vi "LHF.DB.Mongo.Collection.Update.vi"(6 "Query":variant, 8 "error in (no error)":errorcluster, 9 "Update":variant, 10 "Collection":string, 11 "LHF.DB.Mongo in":refnum<class "LHF.DB.Mongo.lvclass">) -> (0 "error out":errorcluster, 1 "DocumentsAffected":i64, 2 "Ok":bool, 3 "LHF.DB.Mongo out":refnum<class "LHF.DB.Mongo.lvclass">)   [LabVIEW 2013, in "LHF.DB.Mongo.lvclass"]
doc: "Update: wire cluster of elements to be updated, use element name to choose database field to update. If a single field being updated you may name the variable name as the desired field to be updated.\nQuery: use clusters named with query operation (if none, equal is used) or a Query.NET object. If a single field is being queried, you may it by setting the variable name as the field name in database. \nYou may use <, <=, >, >=, ==, !=, and others in variables name to choose operation, and you may aggregate them by putting in a cluster with $and or $or."
uses:
  LHF.DB.Mongo.lvclass
  C:/Users/Ricardo/Desktop/Projetos/LabVIEW-MongoDB/src/Driver/MongoDB.Driver.dll
  LabVIEW-MongoDB/src/Driver/MongoDB.Driver.dll
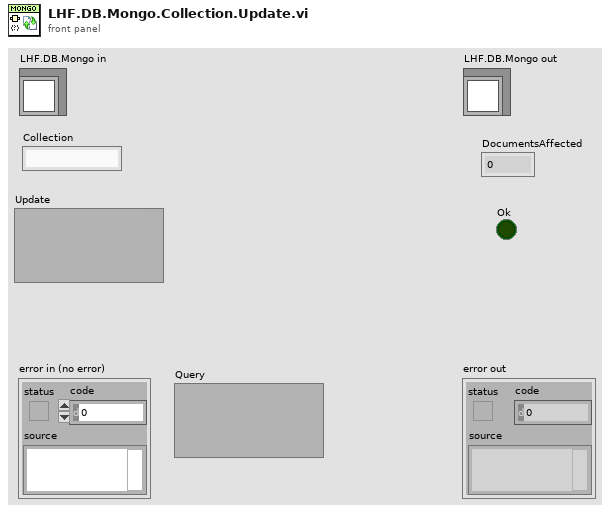
[diagram p1: front panel]
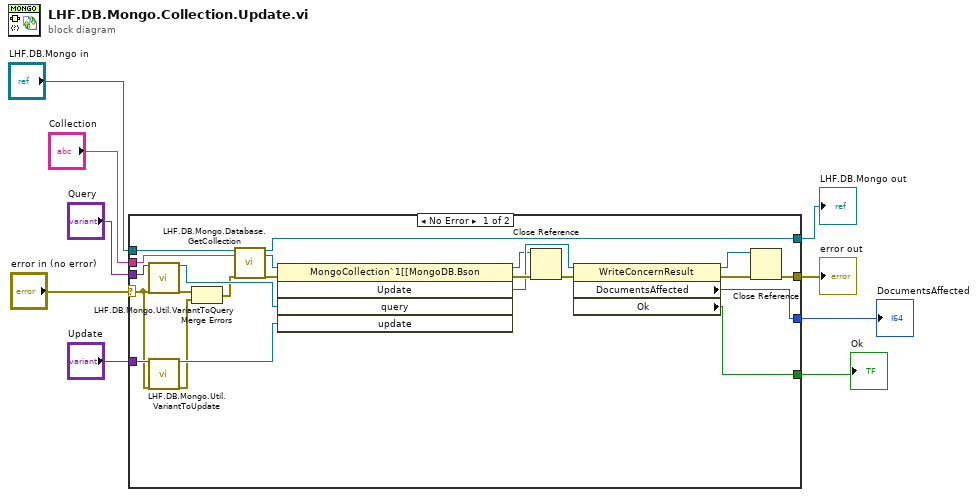
[diagram p0: block diagram]
diagram:
  n1 = case shown="No Error" "error in (no error)" {
    selector: "error in (no error)" -> [w12 w33]
    tunnel: [w13 w33] -> w8
    tunnel: [w23 w32] -> w6
    tunnel: "LHF.DB.Mongo in" -> [w24 w32]
    tunnel: "Collection" -> [w22 _]
    tunnel: "Update" -> [w31 _]
    tunnel: "Query" -> [w28 _]
    tunnel: [w11 _] -> w2
    tunnel: [w10 _] -> w1
    frame No Error {
      n2 = call "LHF.DB.Mongo.Util.VariantToQuery.vi"("Equal"=w28, "error in (no error)"=w12) -> (".NET Refnum out"=w27:refnum<k24>, "error out"=w26:errorcluster)  [unwired: 16 in]
      n3 = call "LHF.DB.Mongo.Util.VariantToUpdate.vi"("Set"=w31, "error in (no error)"=w12) -> (".NET Refnum out"=w30:refnum<k24>, "error out"=w29:errorcluster)  [unwired: 16 in]
      n4 = Merge Errors(w26, w29) -> (w21:errorcluster)
      n5 = call "LHF.DB.Mongo.Database.GetCollection.vi"("LHF.DB.Mongo in"=w24, "collectionName"=w22, "error in (no error)"=w21) -> ("LHF.DB.Mongo in"=w23:refnum<class "LHF.DB.Mongo.lvclass">, "MongoCollection"=w25:refnum<k24>, "error out"=w20:errorcluster)  [unwired: 14 in]
      n6 = invoke class="MongoCollection`1[[MongoDB.Bson" method="Update"(reference=w25, error in=w20, "query"=w27, "update"=w30) -> (reference out=w17:refnum<k24>, error out=w19:errorcluster, "Update"=w18:refnum<k24>)  [unwired: 1 in, 2 out]
      n7 = Close Reference(reference=w17, error in (no error)=w19) -> (error out=w14:errorcluster)
      n8 = property class="WriteConcernResult"(reference=w18, error in=w14) -> (reference out=w16:refnum<k24>, error out=w15:errorcluster, "DocumentsAffected"=w11:i64, "Ok"=w10:bool)
      n9 = Close Reference(reference=w16, error in (no error)=w15) -> (error out=w13:errorcluster)
    }
    frame Error {
    }
  }
  "error out" <- w8
  "LHF.DB.Mongo out" <- w6
  "DocumentsAffected" <- w2
  "Ok" <- w1
